vi "KeyenceCVX.Main-ScanAck.vi"(6 "get img (F)":bool, 7 "TriggerNo":T1 items=["1"=1, "2"=2, "3"=3, "4"=4, "ALL"=5], 8 "error in":errorcluster, 9 "imgpath":path, 11 "Retries (-1: Default)":i32=-1) -> (0 "error out":errorcluster, 2 "CVX Readout details":T5, 3 "CVX Status":T2 {"TriggerNo" items=["1"=1, "2"=2, "3"=3, "4"=4, "ALL"=5]})   [LabVIEW 2016]
uses:
  KeyenceCVX.CodeDetails.ctl
  KeyenceCVX.Data.Status.ctl
  KeyenceCVX.Data.Status.State.ctl
  private/controls/TriggerNo.ctl
  private/controls/RunMode.ctl
  KeyenceCVX.Action.ctl
  KeyenceCVX.ScanAckData.ctl
  tools/EventLog/EventLog.EventSource.ctl
  tools/Translator/Translator.Message.ctl
  tools/EventLog/EventLog.CreateError(array).vi
  tools/Translator/Translator.Translate.Status (NoError).vi
  tools/Translator/Translator.FormatMessage.vi
  tools/EventLog/EventLog.New(array).vi
  Keyence/LowLevel/Keyence.Global.vi
  tools/Translator/Translator.Global.vi
  tools/ErrorHandling/ErrorHandling.Create.vi
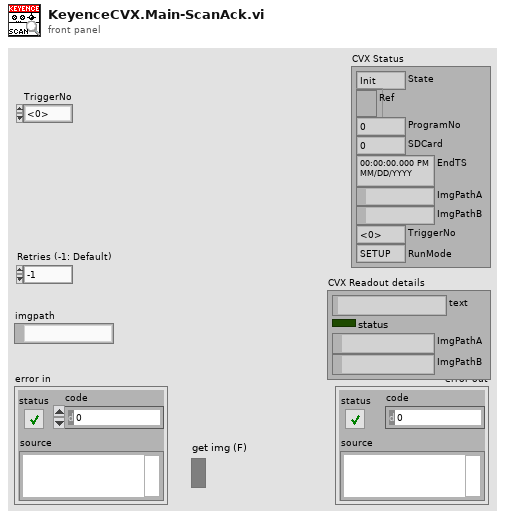
[diagram p1: front panel]
types:
  T1 = typedef "TriggerNo.ctl" = u8
  T2 = typedef "KeyenceCVX.Data.Status.ctl" = cluster{"State":T3, "Ref":refnum<k5>, "ProgramNo":u16, "SDCard":u8, "EndTS":timestamp, "ImgPathA":path, "ImgPathB":path, "TriggerNo":T1, "RunMode":T4}
  T3 = typedef "KeyenceCVX.Data.Status.State.ctl" = enum16{"Init", "Idle", "Scan", "Reset", "ScanAck", "ChangeProgram"}
  T4 = typedef "RunMode.ctl" = enum16{"SETUP", "RUN"}
  T5 = typedef "KeyenceCVX.CodeDetails.ctl" = cluster{"text":string, "status":bool, "ImgPathA":path, "ImgPathB":path}
  T6 = typedef "KeyenceCVX.ScanAckData.ctl" = cluster{"Retries":i32, "ImgPath":path, "ReadImg":bool, "TriggerNo":T1}
  T7 = typedef "KeyenceCVX.Action.ctl" = enum32{"idle", "constructor", "destructor", "-- Keyence CVX --", "Init", "Scan", "ChangeProgram", "ScanAck"}
  T8 = typedef "Translator.Message.ctl" = enum16{"-", "Event confirmed", "Log out", "Log in", "Shutdown", "Cancel", "Start", "Begin time", "End time", "Duration", "Service Mode", "Ignore Results", "Serial Format", "On", "Off", "OK", "NOK", "NOK %s", "Home", "Work", "Close", "Open", "In progress...", "Missing", "Empty", "Hardware failure", "Initial", "Default", "Total", "Out of range", "Free disk space is below 1GB - contact technician", "Error %d >> %s", "Error %d >> %s >> %s", "Msg %d >> %s", "Laser msg %d %s", "Laser cmd error %s %d", "Laser cmd failed %s", "Laser cmd warning %s", "Laser disconnected", "Laser status %s", "Laser already started", "Laser job unkonwn %s", "Laser job missing %s", "Laser job select failure %s", "Unable to start laser printing (%s)", "Unable to stop laser printing (%s)", "Laser marking aborted", "Laser marking timeout", "Unable to reset Laser Interlock (%s)", "Unable to trigger Laser. Laser not ready (%s)", "Laser job '%s' coordinates not configured", "Starting %s", "Quitting %s", "Configured", "Initializing", "Quitting", "Loading", "Loaded %d results", "Loaded %d events", "Running", "Stopped", "Summary", "Laser", "Do you want to continue?", "Do you want to delete the configuration?", "The configuration is being used by an order. Unable to delete!", "Press confirm button", "Station is not based. Do you want to exit?", "Station requires changeover. Do you want to run the test?", "Test options are not set as default. Do you want to continue?", "Formatting of WabcoNo is disabled. Do you want to continue?", "Product not detected. Do you want to continue?", "Product scan failed. Do you want to continue?", "Calibration", "Log out?", "System", "All", "IDLE", "Translating...%s", "Not found", "Alarm %s", "Run", "Skip", "Abort", "Repeat", "Please wait...", "Database disconnected", "Database disconnected - changeover disabled!", "Login to database successful", "Login to database failed: %d; %s", "Unable to check the product status of reference %d - database disconnected", "Unable to set the product status of reference %d - database disconnected", "Variant file backup %s", "Read variant (%s)", "Result", "Station armed!", "Station requires changeover!", "Select reference number...", "EMERGENCY BUTTON - press Control button", "EMERGENCY DOOR - press Control button", "Resetting Emergency...", "Unable to reset safety circuit - Emergency Button pressed", "Unable to reset safety circuit - Emergency Side Door open", "Station not based", "Station based", "Station not empty", "Station basing...", "No order", "Press Start to begin new order", "Scanning new order", "Order NOK. Correct or scan again", "Order OK. Press Accept", "Order ready", "Revolver incorrect", "Fork incorrect", "Revolver missing", "Revolver empty", "Container missing", "Offline results", "Offline statistics", "Updating statistics %.1f %%", "DMC Configurator", "Door open", "Close the front door", "Press start button", "Done. Open the front door", "Running...", "Running...%.1f %%", "Pause %s", "Pause %s. NOK container missing", "Pause %s. OK container missing", "Pause %s. Revolver empty", "Pause %s. Revolver missing", "Pause %s. Revolver incorrect", "Pause %s. Fork missing", "Pause %s. Fork incorrect", "Pause %s. Too many failures", "Pause %s. Unloading failure", "Pause %s. One slot is not working", "Pause %s. Part order is done. Empty OK container", "Pause %s. Unable to move product to slot", "Pause %s. Unable to move back product pusher", "Pause %s. Unable to lift product", "Pause %s. Unable to move back product lifter", "Pause %s. Unable to move product arm to Work", "Pause %s. Unable to move product arm to NOK", "Pause %s. Unable to move product arm to OK", "Pause %s. Unable to unsuck the NOK product", "Pause %s. Unable to drop the NOK product", "Pause %s. Product OK missing", "Pause %s. Unable to unsuck the OK product", "Pause %s. Unable to drop the OK product", "Stopping...", "File '%s' is missing", "File '%s' is broken", "File '%s' is running", "Log file started (%s)", "Log file ended (%s)", "Log file stopped (%s)", "Log file ignored (%s)", "Log file exported (%s)", "Log file export failed (%s)", "Wrong serial number in log file", "Wrong reference number in log file", "Test steps are missing", "%s = %.3f", "Process param '%s' not found in DB", "Process param '%s' wrong order", "Process param '%s' value %.3f out of limits (%.3f; %.3f)", "Step%d param '%s' not found in DB", "Step%d param '%s' wrong order", "Step%d param '%s' value %.3f out of limits (%.3f; %.3f)", "Step%d EV '%s' not found in DB", "Step%d EV '%s' wrong order", "\"%s\" not found in DB", "\"%s\" wrong order", "\"%s\" value %.3f out of limits (%.3f; %.3f)", "\"%s\" not found in software", "Process init (%s)", "Process started", "Process restarted", "Process run", "Process done", "Process done - remove OK container", "Process aborted", "Process aborted at work", "Process aborted at home", "Process error", "Process error at home", "Process error at work", "Process close", "Process pause", "Process continue", "Process door open", "Process door close", "Process pause at slot %s due to %s", "Select plate from the order to process", "Do you want to start the process?", "Do you want to continue the process?", "There is unfinished order. Do you want to put the new order?", "Product %s %d OK", "Product %s %d NOK", "Unable to unload the slot %s. Product missing in the slot", "Unable to unload the slot %s. Product already in the arm", "Unable to accept the product as OK. Product missing in slot %s", "Unable to accept the product as OK. Product could not drop into the container at slot %s", "Unable to accept the product as NOK. Product could not drop into the container at slot %s", "Scan failed. Error %s", "Scan failed. Scanner disconnected", "Scan failed. Wrong Wabco number %d, limit (%d,%d)", "Scan failed. Wrong serial number %d, limit (%d,%d)", "Scan failed. Wrong date %d, limit (%d,%d)", "Scan failed. Wrong product wabco number %d (expected %d)", "Scan failed. Wrong product serial number %d (expected > 0)", "Scan OK %s", "Scan failed. Unable to determine table position (%s)", "Scan failed. Timeout", "Tune failed. Scanner disconnected", "Tune failed. Timeout", "%s = %d", "%s = %d->%d", "Unable to set %s = %.2f - Air Pressure Inside off", "Unable to set digital output '%s' = %d", "Unable to activate air pressure inside - timeout", "Unable to activate air pressure inside - aborted", "Unable to switch on Air Main Valve - Air Pressure Inlet off", "Unable to switch on Air Main Valve - Door open", "Unable to switch off Air Main Valve - timeout", "Unable to switch off Air Main Valve - aborted", "Unable to rotate Table - timeout", "Unable to rotate Table - aborted", "Unable to rotate Table - Product Move not in Home position", "Unable to rotate Table - Air Pressure Inside off", "Unable to rotate Table - Product Lift A not in Home position", "Unable to rotate Table - Product Lift B not in Home position", "Unable to rotate Table - unlock before movement timeout", "Unable to rotate Table - lock after movement timeout", "Unable to move Table Lock to %s position - timeout", "Unable to move Table Lock to %s position - aborted", "Unable to move Table Lock to %s position - Air Pressure Inside off", "Unable to move Table Lock to %s position - Table not in position", "Unable to move Product Lift A to %s position - timeout", "Unable to move Product Lift B to %s position - timeout", "Unable to move Product Lift A to %s position - aborted", "Unable to move Product Lift B to %s position - aborted", "Unable to move Product Lift A to %s position - Air Pressure Inside off", "Unable to move Product Lift B to %s position - Air Pressure Inside off", "Unable to move Product Lift A to %s position - Table not locked", "Unable to move Product Lift B to %s position - Table not locked", "Unable to move Product Lift A to %s position - Product Arm not in Work position", "Unable to move Product Lift B to %s position - Product Arm not in Work position", "Unable to set Product Suction Gripper %s to %s - timeout", "Unable to set Product Suction Gripper %s to %s - aborted", "Unable to set Product Suction Gripper %s to %s - Air Pressure Inside off", "Unable to set Product Suction Gripper %s to %s - Table slot unkown", "Unable to move Product Arm to %s position - timeout", "Unable to move Product Arm to %s position - aborted", "Unable to move Product Arm to %s position - Air Pressure Inside off", "Unable to move Product Arm to %s position - Product Lift A not in Home position", "Unable to move Product Arm to %s position - Product Lift B not in Home position", "Unable to move Product to %s position - timeout", "Unable to move Product to %s position - aborted", "Unable to move Product to %s position - Air Pressure Inside off", "Unable to move Product to %s position - Table not in position"}
  T9 = typedef "EventLog.EventSource.ctl" = enum16{"All", "Gui", "Ref", "File", "Arch", "Seq", "CPX", "DB", "Laser", "Scan.P", "Scan.O"}
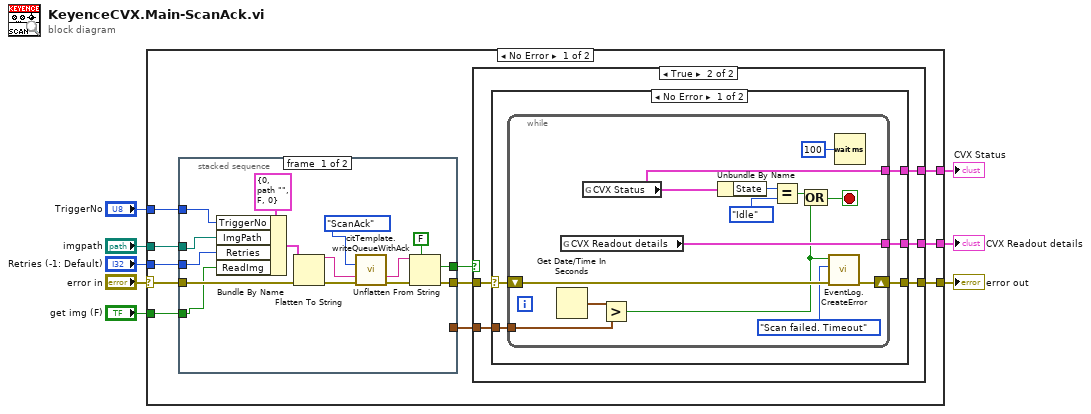
[diagram p0: block diagram]
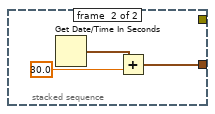
[diagram p2: hidden frame]
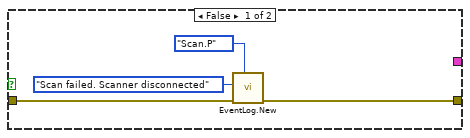
[diagram p3: hidden frame]
diagram:
  n1 = case shown="No Error" "error in" {
    selector: "error in" -> [w19 w66]
    tunnel: [w18 w66] -> w7
    tunnel: [w17 _] -> w3
    tunnel: "imgpath" -> [w13 _]
    tunnel: [w12 _] -> w2
    tunnel: "Retries (-1: Default)" -> [w11 _]
    tunnel: "get img (F)" -> [w10 _]
    tunnel: "TriggerNo" -> [w9 _]
    frame No Error {
      n2 = stacked-sequence {
        tunnel: w19 -> [w34 _]
        tunnel: [w28 _] -> w16
        tunnel: [w27 _] -> w15
        tunnel: [_ w35] -> w14
        tunnel: w13 -> [w24 _]
        tunnel: w11 -> [w23 _]
        tunnel: w10 -> [w22 _]
        tunnel: w9 -> [w21 _]
        frame #0 {
          n3 = Bundle By Name(cluster=T6 {"Retries"=0, "ImgPath"=path "", "ReadImg"=FALSE, "TriggerNo"=0} ("Cluster"), "TriggerNo"=w21, "ImgPath"=w24, "Retries"=w23, "ReadImg"=w22) -> (w20:T6)
          n4 = Flatten To String(anything=w20, error in (no error)=w34) -> (data string=w32:string, error out=w33:errorcluster)  [unwired: 2 in, 1 out]
          n5 = call "citTemplate.writeQueueWithAck.vi"("event in"=KeyenceCVX.Action."ScanAck" ("Action"), "(flatten) data in"=w32, "error in (no error)"=w33) -> ("notification data"=w30:string, "error out"=w31:errorcluster)  [unwired: 10 in, 1 out]
          n6 = Unflatten From String(type=FALSE, binary string=w30, error in (no error)=w31) -> (value=w27:bool, error out=w28:errorcluster)  [unwired: 2 in, 1 out]
        }
        frame #1 {
          n7 = Get Date/Time In Seconds() -> (seconds since 1Jan1904=w37:timestamp)
          n8 = Add(x=w37, y=30.0) -> (x+y=w35:timestamp)
        }
      }
      n9 = case shown="True" w15 {
        tunnel: w16 -> [w40 w46]
        tunnel: [w39 w45] -> w18
        tunnel: [_ w44] -> w17
        tunnel: w14 -> [_ w43]
        tunnel: [_ w42] -> w12
        frame False {
          n10 = call-poly "EventLog.New.vi"("Source (All)"=EventLog.EventSource."Scan.P", "error in (no error)"=w40, "Message (-)"=Translator.Message."Scan failed. Scanner disconnected") -> ("error out"=w39:errorcluster)  [unwired: 7 in, 1 out]
        }
        frame True {
          n11 = case shown="No Error" w46 {
            selector: w46 -> [w50 w65]
            tunnel: [w49 w65] -> w45
            tunnel: [w51 _] -> w44
            tunnel: w43 -> [w48 _]
            tunnel: [w47 _] -> w42
            frame No Error {
              n12 = while {
                tunnel: [w63] -> w51
                shift-right: [w58] -> w49
                shift-left: w50 -> [w62]
                tunnel: w48 -> [w61]
                tunnel: [w55] -> w47
                stop <- w59 stop-if-true
                n13 = Get Date/Time In Seconds() -> (seconds since 1Jan1904=w60:timestamp)
                n14 = global read "Keyence.Global.vi" "CVX Readout details"() -> (w63:T5)
                n15 = global read "Keyence.Global.vi" "CVX Status"() -> (w55:T2)
                n16 = Greater?(x=w60, y=w61) -> (0:w57:bool)
                n17 = Unbundle By Name(w55) -> ("State"=w54:T3)
                n18 = Equal?(x=w54, y=KeyenceCVX.Data.Status.State."Idle" ("State")) -> (x = y?=w52:bool)
                n19 = Compound Arithmetic op=OR(w52, w57) -> (w59:bool)
                n20 = call-poly "EventLog.CreateError.vi"("error in"=w62, "msg"=Translator.Message."Scan failed. Timeout", "create (T)"=w57) -> ("error out"=w58:errorcluster)  [unwired: 7 in, 1 out]
                n21 = Wait (ms)(milliseconds to wait=u32 100) -> ()  [unwired: 1 out]
              }
            }
            frame Error {
            }
          }
        }
      }
    }
    frame Error {
    }
  }
  "error out" <- w7
  "CVX Readout details" <- w3
  "CVX Status" <- w2
